vi "Close SC2250 Sessions And Clear Cache.vi"(11 "error in (no error)":errorcluster) -> (15 "error out":errorcluster)   [LabVIEW 2023, in "RFFixtureCharact.RFPM.lvlib" / "SG SC2250 Path Group.lvclass"]
uses:
  SG SC2250 Path Group.lvclass
  Common/Data Cache/Type Definitions/Dictionary Operation.ctl
  Common/RFCalAndFixtureCharact.Common.lvlib
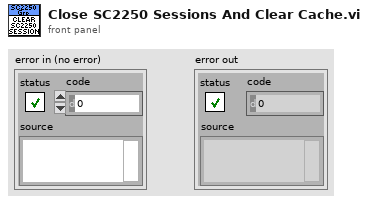
[diagram p1: front panel]
types:
  T1 = typedef "RFCalAndFixtureCharact.Common.lvlib/Dictionary Operation.ctl" = enum16{"Read", "Insert", "Remove", "Clear", "Get All", "Update"}
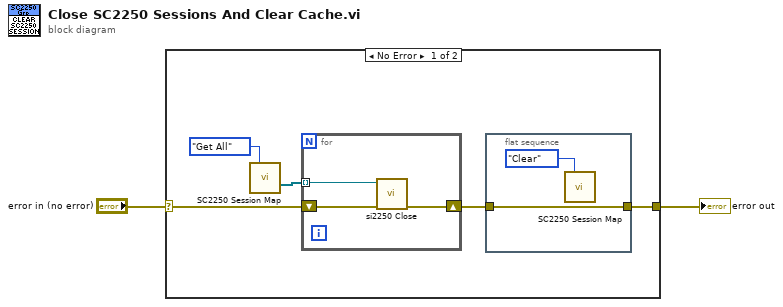
[diagram p0: block diagram]
diagram:
  n1 = case shown="No Error" "error in (no error)" {
    selector: "error in (no error)" -> [w5 w13]
    tunnel: [w4 w13] -> w1
    frame No Error {
      n2 = call "SC2250 Session Map.vi"("Action"=Dictionary_Operation."Get All") -> ("sc2250 sessions"=w6:refnum<k15>[])  [unwired: 12 in, 2 out]
      n3 = for {
        tunnel: w6 -> [w12] mode=indexing
        shift-right: [w10] -> w3
        shift-left: w5 -> [w11]
        n4 = call <instrlib>:"si2250 Close.vi"("error in"=w11, "instrument handle"=w12) -> ("error out"=w10:errorcluster)  [unwired: 9 in]
      }
      n5 = flat-sequence {
        tunnel: [w8] -> w4
        tunnel: w3 -> [w8]
        frame #0 {
          n6 = call "SC2250 Session Map.vi"("Action"=Dictionary_Operation."Clear") -> ()  [unwired: 12 in, 3 out]
        }
      }
    }
    frame Error {
    }
  }
  "error out" <- w1
